vi "1-Wire.vi"(4 "1-Wire":T1={"SENS"=11, "DPU"=0, "Options"=0, "Function"=0, "Num Tx"=0, "Num Rx"=0, "TX Data"=[], "ROM H"=0, "ROM L"=0, "Branches H"=0, "Branches L"=0, "Search Res H"=0, "Search Res L"=0, "Path H"=0, "Path L"=0} {"Path L" format="%x"; "Path H" format="%x"; "Search Res L" format="%x"; "Search Res H" format="%x"; "Branches L" format="%x"; "Branches H" format="%x"; "ROM L" format="%x"; "ROM H" format="%x"; "TX Data" format="%x"; "Function" format="%x"}, 5 "Identifier":string="LJM_idANY", 6 "ConnectionType":string="LJM_ctANY", 7 "DeviceType":string="LJM_dtANY") -> (0 "Error String":string, 1 "error out":errorcluster, 2 "aData":u32[](array[numeric]) format="%x", 3 "aValuesOut":u32[](array[numeric]) format="%x")   [LabVIEW 2020]
panel:
  in  "Case Constant\n(See Context Help)":bool=TRUE
  # "Functions: \nSearch 0xF0\nSkip 0xCC\nMatch 0x55\nRead 0x33"
  # "Searching for a 1-Wire Probe ROM Id:\n1. Configure SENS channel,\n    0: FIO0\n    1: FIO1\n    8: EIO0\n    9: EIO1\n    10: EIO2\n    11: EIO3\n    12: EIO4\n    13: EIO5\n    14: EIO6\n    15: EIO7\n     etc.\n2. Set the \"Functions\" option to 0xF0\n3. Run the .vi\n4. \"ROM H\" reports the upper bytes and \n    \"ROM L\" reports the lower bytes of the \n    1-wire chip ID."
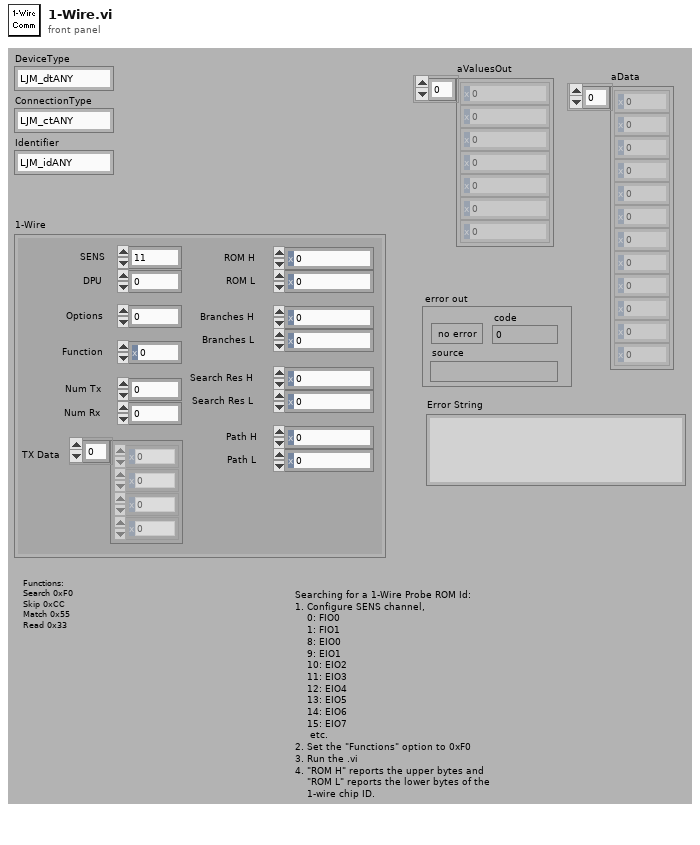
[diagram p1: front panel]
types:
  T1 = cluster{"SENS":u32, "DPU":u32, "Options":u32, "Function":u32, "Num Tx":u32, "Num Rx":u32, "TX Data":u16[], "ROM H":u32, "ROM L":u32, "Branches H":u32, "Branches L":u32, "Search Res H":u32, "Search Res L":u32, "Path H":u32, "Path L":u32}
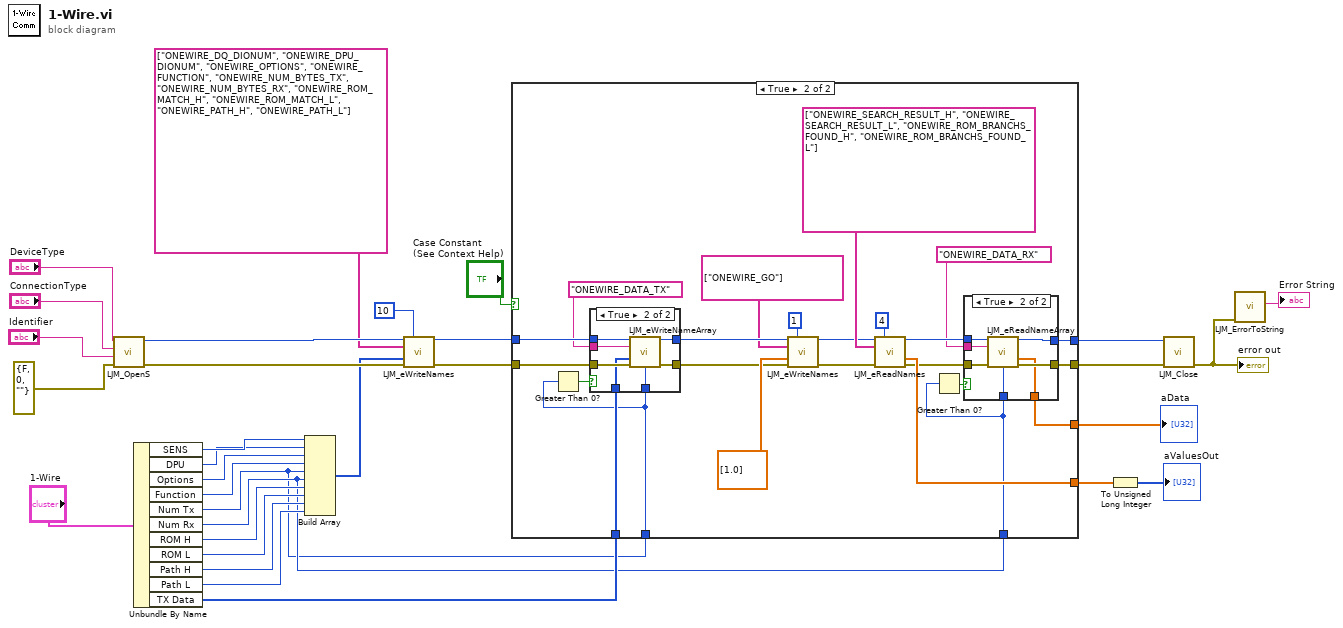
[diagram p0: block diagram]
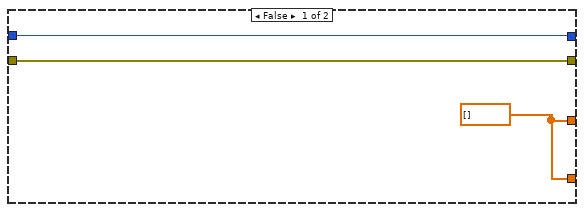
[diagram p2: hidden frame]
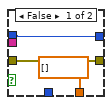
[diagram p3: hidden frame]
diagram:
  n1 = call "LJM_OpenS.vi"("error in"=errorcluster {"status"=FALSE, "code"=0, "source"=""} ("error in (no error)"), "Identifier"="Identifier", "ConnectionType"="ConnectionType", "DeviceType"="DeviceType") -> ("error out"=w25:errorcluster, "Handle"=w24:i32)  [unwired: 6 in]
  n2 = Unbundle By Name("1-Wire") -> ("SENS"=w20:u32, "DPU"=w19:u32, "Options"=w18:u32, "Function"=w17:u32, "Num Tx"=w1:u32, "Num Rx"=w3:u32, "ROM H"=w16:u32, "ROM L"=w15:u32, "Path H"=w14:u32, "Path L"=w13:u32, "TX Data"=w4:u16[])
  n3 = Build Array(w20, w19, w18, w17, w1, w3, w16, w15, w14, w13) -> (w12:u32[])
  n4 = call "LJM_eWriteNames.vi"("Handle In"=w24, "NumFrames (Auto-Detect)"=10 ("NumFrames"), "aNames"=string[] ["ONEWIRE_DQ_DIONUM", "ONEWIRE_DPU_DIONUM", "ONEWIRE_OPTIONS", "ONEWIRE_FUNCTION", "ONEWIRE_NUM_BYTES_TX", "ONEWIRE_NUM_BYTES_RX", "ONEWIRE_ROM_MATCH_H", "ONEWIRE_ROM_MATCH_L", "ONEWIRE_PATH_H", "ONEWIRE_PATH_L"], "aValuesIn"=w12, "error in"=w25) -> ("Handle Out"=w8:i32, "error out"=w11:errorcluster)  [unwired: 8 in, 1 out]
  n5 = case shown="True" "Case Constant\n(See Context Help)" {
    tunnel: w11 -> [w33 w49]
    tunnel: [w33 w43] -> w10
    tunnel: [w34 w44] -> w9
    tunnel: w8 -> [w34 w48]
    tunnel: [w32 w56] -> w5
    tunnel: w4 -> [_ w40]
    tunnel: w3 -> [_ w35]
    tunnel: [w32 w41] -> w2
    tunnel: w1 -> [_ w37]
    frame False {
      w32 = dbl[] [] ("aValuesOut")
    }
    frame True {
      n6 = Greater Than 0?(x=w37) -> (x > 0?=w38:bool)
      n7 = case shown="True" w38 {
        tunnel: w49 -> [w69 w74]
        tunnel: [w69 w77] -> w47
        tunnel: [w70 w76] -> w55
        tunnel: w48 -> [w70 w75]
        tunnel: w37 -> [_ w73]
        tunnel: w40 -> [_ w72]
        tunnel: "ONEWIRE_DATA_TX" ("String") -> [_ w71]
        frame False {
        }
        frame True {
          n8 = call "LJM_eWriteNameArray.vi"("Handle In"=w75, "Name"=w71, "aValues"=w72, "error in"=w74, "NumValues"=w73) -> ("Handle Out"=w76:i32, "error out"=w77:errorcluster)  [unwired: 8 in, 1 out]
        }
      }
      n9 = call "LJM_eWriteNames.vi"("Handle In"=w55, "NumFrames (Auto-Detect)"=1 ("NumFrames"), "aNames"=string[] ["ONEWIRE_GO"], "aValuesIn"=dbl[] [1.0], "error in"=w47) -> ("Handle Out"=w53:i32, "error out"=w54:errorcluster)  [unwired: 8 in, 1 out]
      n10 = call "LJM_eReadNames.vi"("Handle In"=w53, "NumFrames (Auto-Detect)"=4 ("NumFrames"), "aNames"=string[] ["ONEWIRE_SEARCH_RESULT_H", "ONEWIRE_SEARCH_RESULT_L", "ONEWIRE_ROM_BRANCHS_FOUND_H", "ONEWIRE_ROM_BRANCHS_FOUND_L"], "error in"=w54) -> ("Handle Out"=w45:i32, "aValuesOut"=w56:dbl[], "error out"=w46:errorcluster)  [unwired: 8 in, 1 out]
      n11 = Greater Than 0?(x=w35) -> (x > 0?=w36:bool)
      n12 = case shown="True" w36 {
        tunnel: w46 -> [w60 w68]
        tunnel: w45 -> [w61 w67]
        tunnel: [w61 w66] -> w44
        tunnel: [w60 w65] -> w43
        tunnel: "ONEWIRE_DATA_RX" ("String") -> [_ w64]
        tunnel: w35 -> [_ w62]
        tunnel: [dbl[] [] ("aValues") w63] -> w41
        frame False {
        }
        frame True {
          n13 = call "LJM_eReadNameArray.vi"("Handle In"=w67, "Name"=w64, "error in"=w68, "NumValues"=w62) -> ("Handle Out"=w66:i32, "aValues"=w63:dbl[], "error out"=w65:errorcluster)  [unwired: 8 in, 1 out]
        }
      }
    }
  }
  "aData" <- w2
  n14 = To Unsigned Long Integer(number=w5) -> (unsigned 32bit integer=→"aValuesOut":u32[])
  n15 = call "LJM_Close.vi"("error in"=w10, "Handle"=w9) -> ("error out"=w31:errorcluster)  [unwired: 9 in]
  "error out" <- w31
  n16 = call "LJM_ErrorToString.vi"("error in"=w31) -> ("String"=→"Error String":string)  [unwired: 10 in]
